vi "Hyperterminal.vi"() -> ()   [LabVIEW 2014, in "AD4212C Lib.lvlib"]
doc: "Use this template to build a producer/consumer design pattern with events to produce queue items. Use this design pattern instead of the User Interface Event Handler pattern for user interfaces when you want to execute code asynchronously in response to an event without slowing the user interface responsiveness."
uses:
  AD4212C Lib.lvlib
  States.ctl
  Typedef/Connection Data.ctl
panel:
  out "VISA resource name Out":T1={"Conection Data"="COM4"}
  out "error out":errorcluster
  in  "VISA resource name In":T1={"Conection Data"="COM4"}
  in  "error in (no error)":errorcluster
  out "Value":dbl format="%#_8f"
  in  "Stop":bool
  in  "Initialize":bool
  in  "AutoZero":bool
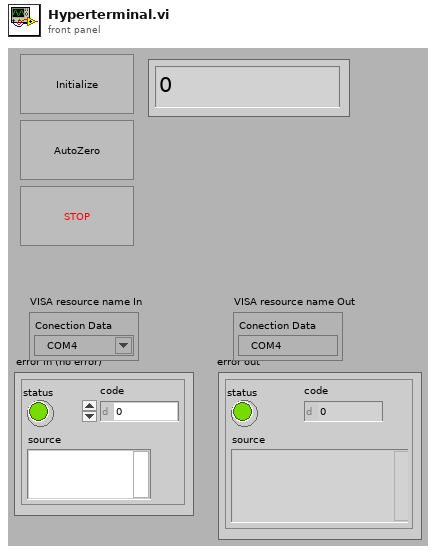
[diagram p1: front panel]
types:
  T1 = typedef "AD4212C Lib.lvlib/Connection Data.ctl" = cluster{"Conection Data":refnum<visa-resource-name>}
  T2 = typedef "AD4212C Lib.lvlib/States.ctl" = enum16{"Wait", "Initialize", "Read Port", "Write Port", "Close"}
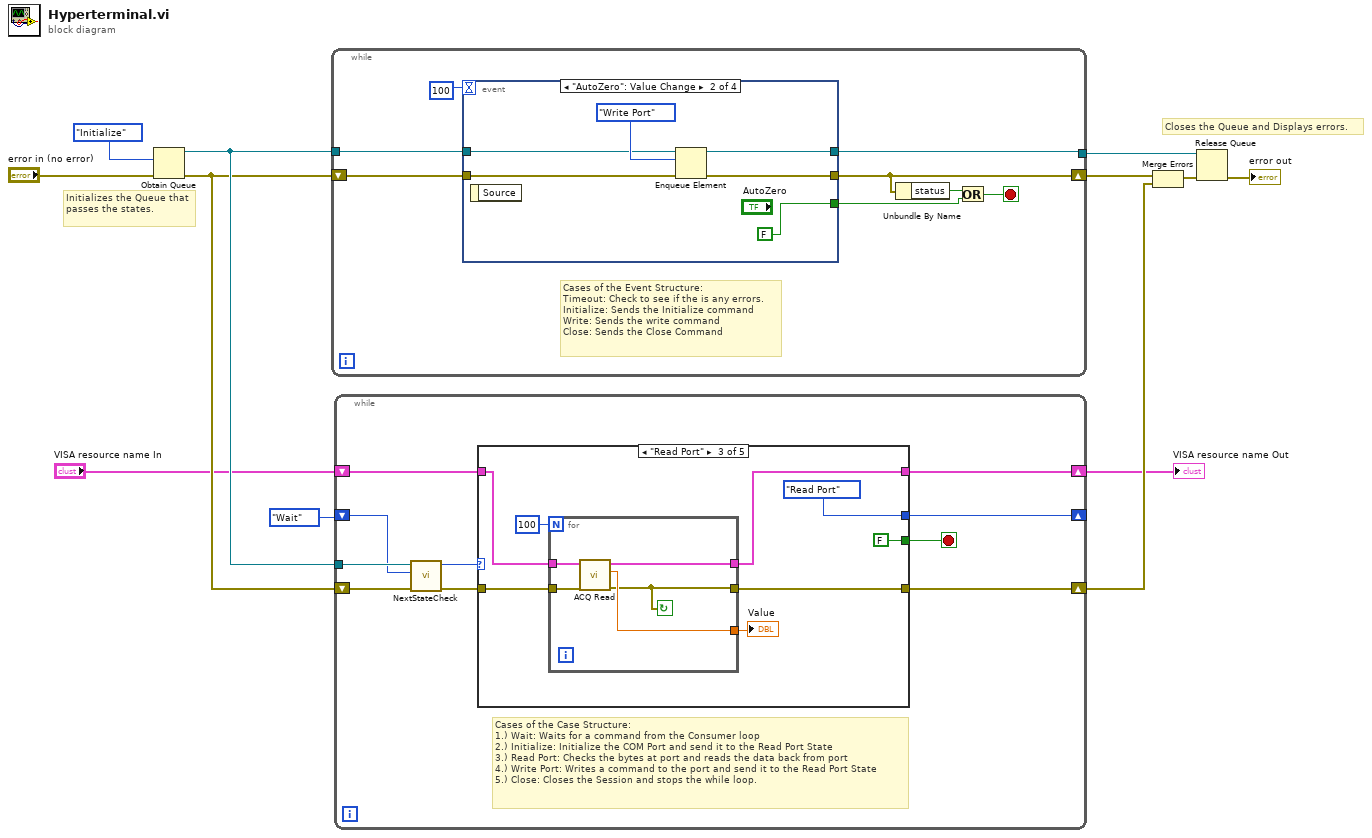
[diagram p0: block diagram]
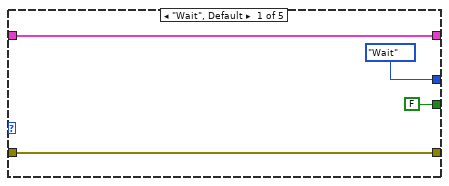
[diagram p2: hidden frame]
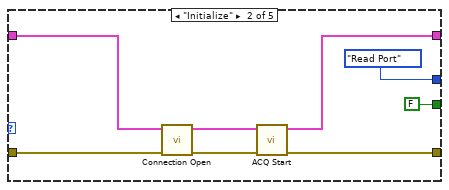
[diagram p3: hidden frame]
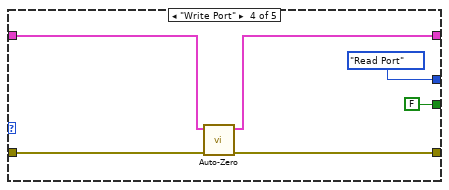
[diagram p4: hidden frame]
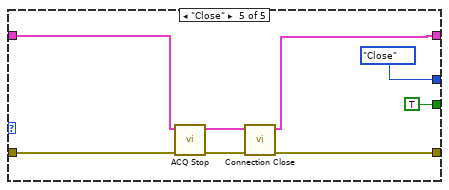
[diagram p5: hidden frame]
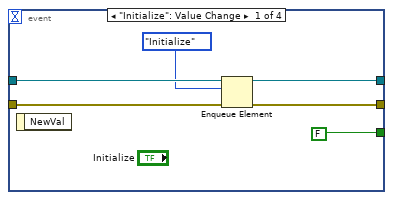
[diagram p6: hidden frame]
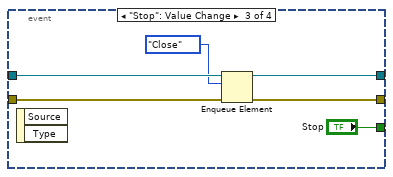
[diagram p7: hidden frame]
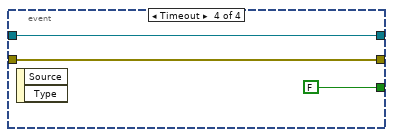
[diagram p8: hidden frame]
diagram:
  # "Closes the Queue and Displays errors."
  # "Initializes the Queue that passes the states."
  n1 = Obtain Queue(element data type=States."Initialize" ("Enum"), error in (no error)="error in (no error)") -> (queue out=w10:refnum<queue>, error out=w8:errorcluster)  [unwired: 3 in, 1 out]
  n2 = while {
    shift-right: [w17] -> w7
    shift-left: w8 -> [w19]
    tunnel: w10 -> [w20]
    tunnel: [w13] -> w5
    stop <- w18 stop-if-true
    # "Cases of the Event Structure:\nTimeout: Check to see if the is any errors.\nInitialize: Sends the Initialize command\nWrite: Sends the write command\nClose: Sends the Close Command"
    n3 = event shown="[1] \"AutoZero\": Value Change" {
      selector: _ -> [_ _ _ _]
      dyn-events: _ -> [_ _ _ _]
      timeout: 100 -> [_ _ _ _]
      tunnel: w20 -> [w26 w31 w35 w39]
      tunnel: w19 -> [w25 w30 w37 w41]
      tunnel: [w23 w29 w36 w41] -> w17
      tunnel: [FALSE ("Stop") FALSE ("Stop") "Stop" FALSE ("Stop")] -> w14
      tunnel: [w21 w27 w33 w39] -> w13
      event "Initialize": Value Change {
        n4 = event-data() -> ()  [unwired: 1 in, 1 out]
        n5 = Enqueue Element(queue=w26, element=States."Initialize", error in (no error)=w25) -> (queue out=w21:refnum<queue>, error out=w23:errorcluster)  [unwired: 1 in, 1 out]
      }
      event "AutoZero": Value Change {
        n6 = event-data() -> ()  [unwired: 1 in, 1 out]
        n7 = Enqueue Element(queue=w31, element=States."Write Port", error in (no error)=w30) -> (queue out=w27:refnum<queue>, error out=w29:errorcluster)  [unwired: 1 in, 1 out]
      }
      event "Stop": Value Change {
        n8 = event-data() -> ()  [unwired: 1 in, 2 out]
        n9 = Enqueue Element(queue=w35, element=States."Close", error in (no error)=w37) -> (queue out=w33:refnum<queue>, error out=w36:errorcluster)  [unwired: 1 in, 1 out]
      }
      event Timeout {
        n10 = event-data() -> ()  [unwired: 1 in, 2 out]
      }
    }
    n11 = Unbundle By Name(w17) -> ("status"=w16:bool)
    n12 = Or(x=w16, y=w14) -> (x .or. y?=w18:bool)
  }
  n13 = while {
    shift-right: [w51] -> w3
    shift-left: "VISA resource name In" -> [w50]
    shift-right: [w42] -> w6
    shift-left: w8 -> [w47]
    shift-right: [w48] -> _
    shift-left: States."Wait" ("Enum") -> [w45]
    tunnel: w10 -> [w46]
    stop <- w49 stop-if-true
    # "Cases of the Case Structure:\n1.) Wait: Waits for a command from the Consumer loop\n2.) Initialize: Initialize the COM Port and send it to the Read Port State\n3.) Read Port: Checks the bytes at port and reads the data back from port\n4.) Write Port: Writes a command to the port and send it to the Read Port State\n5.) Close: Closes the Session and stops the while loop."
    n14 = call "NextStateCheck.vi"("Error In"=w47, "Current State"=w45, "Queue"=w46) -> ("Error Out"=w43:errorcluster, "Checked State"=w44:T2)  [unwired: 7 in]
    n15 = case shown="\"Read Port\"" w44 {
      tunnel: [w55 w59 w68 w79 w87] -> w51
      tunnel: [w52 w58 w64 w78 w88] -> w42
      tunnel: w50 -> [w55 w61 w69 w80 w86]
      tunnel: [States."Wait" ("Enum") States."Read Port" ("Enum") States."Read Port" ("Enum") States."Read Port" ("Enum") States."Close" ("Enum")] -> w48
      tunnel: [FALSE FALSE FALSE FALSE TRUE] -> w49
      tunnel: w43 -> [w52 w56 w67 w77 w83]
      frame "Wait", Default {
      }
      frame "Initialize" {
        n16 = call "Connection Open.vi"("VISA resource name Out 3"=w61, "error in (no error)"=w56) -> ("VISA resource name Out 2"=w60:T1, "error out"=w57:errorcluster)  [unwired: 7 in]
        n17 = call "ACQ Start.vi"("error in (no error)"=w57, "VISA resource name In"=w60) -> ("error out"=w58:errorcluster, "VISA resource name Out"=w59:T1)  [unwired: 8 in]
      }
      frame "Read Port" {
        n18 = for {
          N: 100 -> [_]
          tunnel: [w73] -> w65
          tunnel: w69 -> [w76]
          tunnel: [w75] -> w68
          tunnel: w67 -> [w74]
          tunnel: [w72] -> w64
          stop <- w72 continue-if-true
          n19 = call "ACQ Read.vi"("error in (no error)"=w74, "VISA resource name In"=w76) -> ("error out"=w72:errorcluster, "Value"=w73:sgl, "VISA resource name Out"=w75:T1)  [unwired: 7 in]
        }
        "Value" <- w65
      }
      frame "Write Port" {
        n20 = call "Auto-Zero.vi"("error in (no error)"=w77, "VISA resource name In"=w80) -> ("error out"=w78:errorcluster, "VISA resource name Out"=w79:T1)  [unwired: 8 in]
      }
      frame "Close" {
        n21 = call "ACQ Stop.vi"("error in (no error)"=w83, "VISA resource name In"=w86) -> ("error out"=w84:errorcluster, "VISA resource name Out"=w85:T1)  [unwired: 8 in]
        n22 = call "Connection Close.vi"("error in (no error)"=w84, "VISA resource name In"=w85) -> ("error out"=w88:errorcluster, "VISA resource name Out"=w87:T1)  [unwired: 8 in]
      }
    }
  }
  "VISA resource name Out" <- w3
  n23 = Merge Errors(w7, w6) -> (w9:errorcluster)
  n24 = Release Queue(queue=w5, error in (no error)=w9) -> (error out=→"error out":errorcluster)  [unwired: 1 in, 2 out]
